vi "TildaPassiveTest.vi"() -> ()   [LabVIEW 2014]
uses:
  <vilib>/FPGAPlugInAG/PXI-7852R/niLvFpga_Open_PXI-7852R.vi
  <vilib>/rvi/interface/common/dynamic/niFpgaDynamicAddResources.vi
  <vilib>/Utility/error.llb/Error Cluster From Error Code.vi
  <vilib>/rvi/errors/niLvFpgaAdjustHostInterfaceError.vi
  <vilib>/FPGAPlugInAG/Dynamic/niLvFpga_Close_Dynamic.vi
  <vilib>/rvi/interface/nirviOpenFPGA/nirviOpenFPGA.xnode
  FPGA Bitfiles/TildaPassiveMain_V100.lvbitx
  <vilib>/rvi/interface/nirviReadWriteControl/nirviReadWriteControl.xnode
  <vilib>/rvi/interface/nirviMethod/nirviMethod.xnode
  <vilib>/rvi/interface/nirviCloseFPGA/nirviCloseFPGA.xnode
  <vilib>/rvi/interface/Simulation/niFpgaSimulationCallBeginRW.vi
  NiFpgaLv.dll
  <vilib>/FPGAPlugInAG/Dynamic/niLvFpga_ReadFifo_Dynamic.vi
  <vilib>/rvi/errors/niLvFpgaMergeErrorWithErrorCode.vi
panel:
  out "nOfSteps":u32
  out "nOfScans":u32
  out "counts":u32
  out "saved elements":i32
  in  "delay_10ns_ticks":u32
  in  "nOfBins":u32
  in  "AnalyseData":bool
  out "ReadData":u32[](array[numeric]) format="%032b"
  out "SavedData":u32[](array[numeric]) format="%032b"
  in  "stop":bool
  in  "Start":bool
  out "TildaPassiveStateInd":enum16{"idle", "scanning", "error"}(ring)
  out "error out":errorcluster
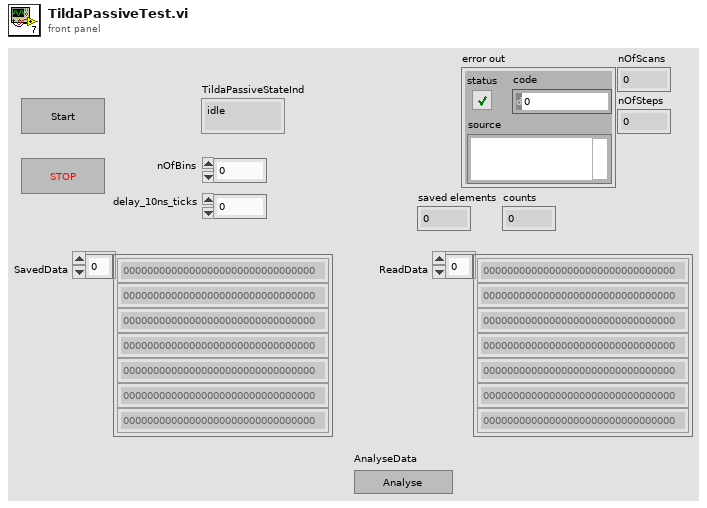
[diagram p1: front panel]
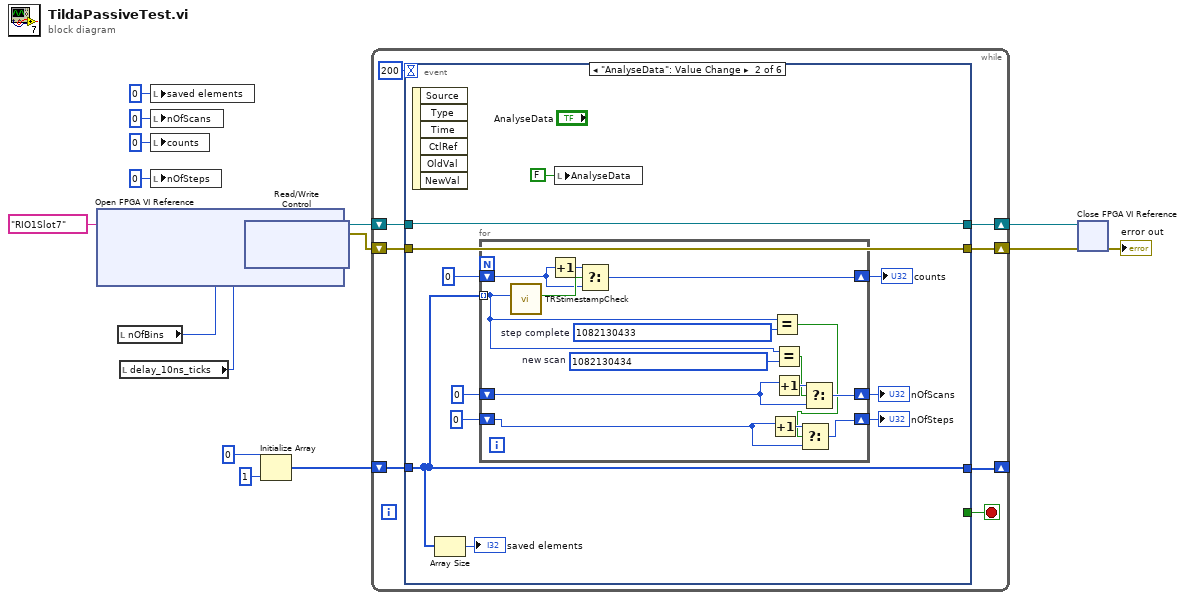
[diagram p0: block diagram]
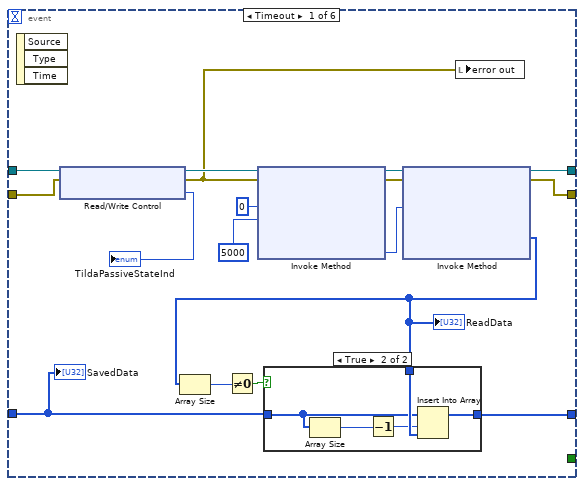
[diagram p2: hidden frame]
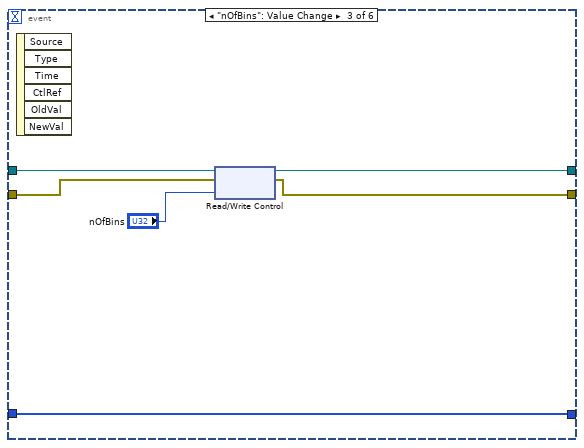
[diagram p4: hidden frame]
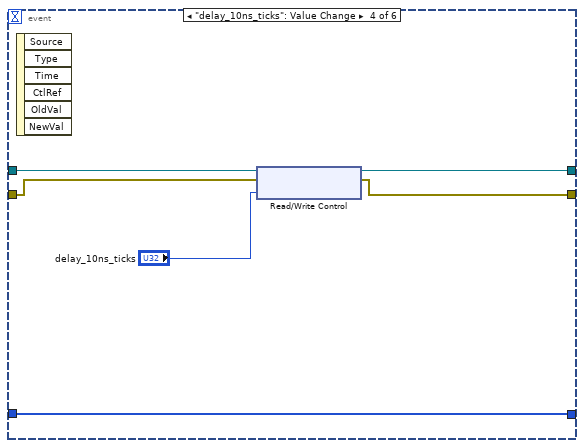
[diagram p5: hidden frame]
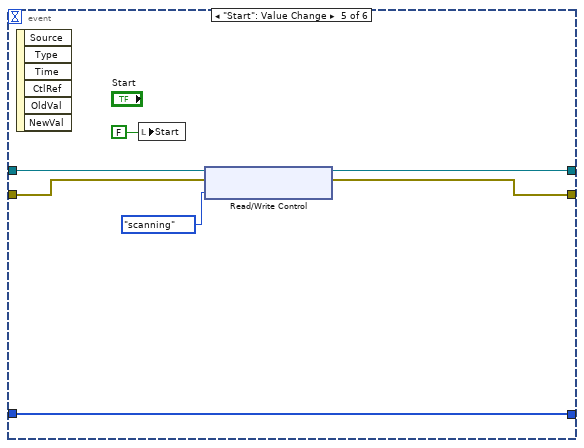
[diagram p6: hidden frame]
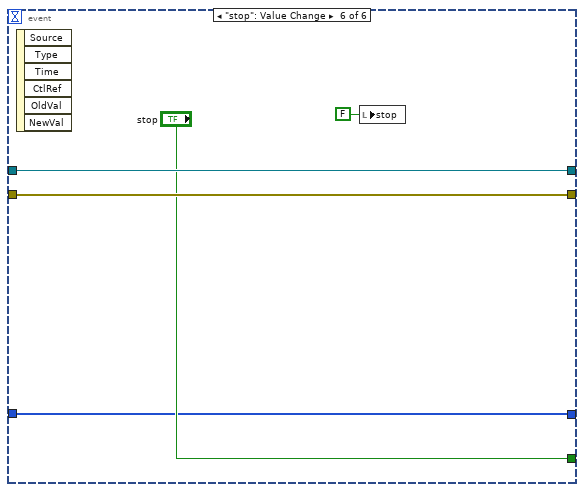
[diagram p7: hidden frame]
diagram:
  n1 = xnode "Open FPGA VI Reference"("resource name"=tag "RIO1Slot7") -> ("FPGA VI Reference Out"=w5:refnum<k20>, "error out"=w4:errorcluster)  [unwired: 1 in]
  n2 = local read "nOfBins"() -> (w12:u32)
  n3 = local read "delay_10ns_ticks"() -> (w11:u32)
  n4 = local write "saved elements"(0 ("saved elements")) -> ()
  n5 = local write "nOfScans"(u32 0 ("nOfScans")) -> ()
  n6 = local write "counts"(u32 0 ("counts")) -> ()
  n7 = local write "nOfSteps"(u32 0 ("nOfSteps")) -> ()
  n8 = xnode "Read/Write Control"("FPGA VI Reference In"=w5, "error in"=w4, "nOfBins"=w12, "delay_10ns_ticks"=w11) -> ("FPGA VI Reference Out"=w3:refnum<k20>, "error out"=w2:errorcluster)
  n9 = Initialize Array(u32 0 ("element"), 1 ("dimension size")) -> (w6:u32[])
  n10 = while {
    shift-right: [w23] -> w17
    shift-left: w3 -> [w24]
    shift-right: [w22] -> w15
    shift-left: w2 -> [w21]
    shift-right: [w19] -> _
    shift-left: w6 -> [w18]
    stop <- w20 stop-if-true
    n11 = event shown="[1] \"AnalyseData\": Value Change" {
      selector: _ -> [_ _ _ _ _ _]
      dyn-events: _ -> [_ _ _ _ _ _]
      timeout: 200 -> [_ _ _ _ _ _]
      tunnel: w24 -> [w42 w57 w80 w86 w93 w98]
      tunnel: [w35 w57 w79 w85 w92 w98] -> w23
      tunnel: [w32 w56 w77 w82 w91 w97] -> w22
      tunnel: w21 -> [w39 w56 w78 w83 w89 w97]
      tunnel: [_ _ _ _ _ "stop"] -> w20
      tunnel: [w28 w53 w75 w81 w88 w95] -> w19
      tunnel: w18 -> [w26 w53 w75 w81 w88 w95]
      event Timeout {
        n12 = event-data() -> ()  [unwired: 1 in, 3 out]
        n13 = xnode "Read/Write Control"("FPGA VI Reference In"=w42, "error in"=w39) -> ("FPGA VI Reference Out"=w41:refnum<k20>, "error out"=w34:errorcluster, "TildaPassiveStateInd"=→"TildaPassiveStateInd":enum16{"idle", "scanning", "error"})
        n14 = xnode "Invoke Method"("FPGA VI Reference In"=w41, "error in"=w34, "Number of Elements"=u32 0, "Timeout (ms)"=5000) -> ("FPGA VI Reference Out"=w38:refnum<k20>, "error out"=w33:errorcluster, "Elements Remaining"=w31:u32)  [unwired: 1 out]
        n15 = xnode "Invoke Method"("FPGA VI Reference In"=w38, "error in"=w33, "Number of Elements"=w31) -> ("FPGA VI Reference Out"=w35:refnum<k20>, "error out"=w32:errorcluster, "Data"=w27:u32[])  [unwired: 1 in, 1 out]
        "ReadData" <- w27
        n16 = Array Size(array=w27) -> (size(s)=w29:i32)
        n17 = Not Equal To 0?(x=w29) -> (x != 0?=w30:bool)
        n18 = case shown="True" w30 {
          tunnel: w27 -> [_ w48]
          tunnel: [w43 w47] -> w28
          tunnel: w26 -> [w43 w46]
          frame False {
          }
          frame True {
            n19 = Array Size(array=w46) -> (size(s)=w45:i32)
            n20 = Decrement(x=w45) -> (x-1=w44:i32)
            n21 = Insert Into Array(array=w46, index=w44, new element=w48) -> (w47:u32[])
          }
        }
        n22 = local write "error out"(w34) -> ()
        "SavedData" <- w26
      }
      event "AnalyseData": Value Change {
        n23 = event-data() -> ()  [unwired: 1 in, 6 out]
        n24 = Array Size(array=w53) -> (size(s)=→"saved elements":i32)
        n25 = for {
          tunnel: w53 -> [w67] mode=indexing
          shift-right: [w73] -> w54
          shift-left: u32 0 ("element") -> [w72]
          shift-right: [w64] -> w51
          shift-left: u32 0 ("element") -> [w65]
          shift-right: [w61] -> w49
          shift-left: u32 0 ("element") -> [w62]
          w69 = u32 1082130434  # new scan
          w70 = u32 1082130433  # step complete
          n26 = call "TRStimestampCheck.vi"("element"=w67) -> ("TRSTimestamp?"=w74:bool)  [unwired: 10 in]
          n27 = Increment(x=w72) -> (x+1=w71:u32)
          n28 = Select(t=w71, s=w74, f=w72) -> (s? t:f=w73:u32)
          n29 = Increment(x=w62) -> (x+1=w63:u32)
          n30 = Equal?(x=w67, y=w70) -> (x = y?=w60:bool)
          n31 = Equal?(x=w67, y=w69) -> (x = y?=w66:bool)
          n32 = Increment(x=w65) -> (x+1=w68:u32)
          n33 = Select(t=w63, s=w60, f=w62) -> (s? t:f=w61:u32)
          n34 = Select(t=w68, s=w66, f=w65) -> (s? t:f=w64:u32)
        }
        "counts" <- w54
        "nOfScans" <- w51
        "nOfSteps" <- w49
        n35 = local write "AnalyseData"(FALSE ("AnalyseData")) -> ()
      }
      event "nOfBins": Value Change {
        n36 = event-data() -> ()  [unwired: 1 in, 6 out]
        n37 = xnode "Read/Write Control"("FPGA VI Reference In"=w80, "error in"=w78, "nOfBins"="nOfBins") -> ("FPGA VI Reference Out"=w79:refnum<k20>, "error out"=w77:errorcluster)
      }
      event "delay_10ns_ticks": Value Change {
        n38 = event-data() -> ()  [unwired: 1 in, 6 out]
        n39 = xnode "Read/Write Control"("FPGA VI Reference In"=w86, "error in"=w83, "delay_10ns_ticks"="delay_10ns_ticks") -> ("FPGA VI Reference Out"=w85:refnum<k20>, "error out"=w82:errorcluster)
      }
      event "Start": Value Change {
        n40 = event-data() -> ()  [unwired: 1 in, 6 out]
        n41 = local write "Start"(FALSE ("Start")) -> ()
        n42 = xnode "Read/Write Control"("FPGA VI Reference In"=w93, "error in"=w89, "TildaPassiveStateCtrl"=enum16{"idle", "scanning", "error"}."scanning") -> ("FPGA VI Reference Out"=w92:refnum<k20>, "error out"=w91:errorcluster)
      }
      event "stop": Value Change {
        n43 = event-data() -> ()  [unwired: 1 in, 6 out]
        n44 = local write "stop"(FALSE ("stop")) -> ()
      }
    }
  }
  n45 = xnode "Close FPGA VI Reference"("FPGA VI Reference In"=w17, "error in"=w15) -> ("error out"=→"error out":errorcluster)
